vi "SetNag_record_pressure_and_temp.vi"() -> ()   [LabVIEW 2013]
uses:
  <vilib>/Utility/file.llb/Write To Spreadsheet File (string).vi
  <vilib>/Utility/file.llb/Write To Spreadsheet File (DBL).vi
panel:
  out "Read 6":string
  in  "Write 6":string="_STP\r"
  out "Waveform Chart 2":T1(graph)
  out "Read 5":string
  in  "Write 5":string="_TEM\r"
  in  "Write 4":string="_AMB\r"
  out "Read 4":string
  in  "milliseconds to wait":u32=100
  in  "Write 1":string="_OXY\r"
  out "Read 3":string
  in  "Write 3":string="_ETA\r"
  in  "stop 2":bool
  out "Read 2":string
  in  "Write 2":string="_PAB\r"
  out "Read 1":string
  out "Waveform Chart":T2(graph)
  in  "Com Port":i32(ring) items=["Com 1", "Com 2", "Com 3", "Com 4", "Com 5", "Com 6", "COM 7", "COM 8", "COM 9", "COM 10", "COM 11", "COM 12", "com 13", "COM 14"]
  in  "Baud Rate":i32(ring)=2 items=["2400", "4800", "9600", "19200", "38400", "57600", "115200"]
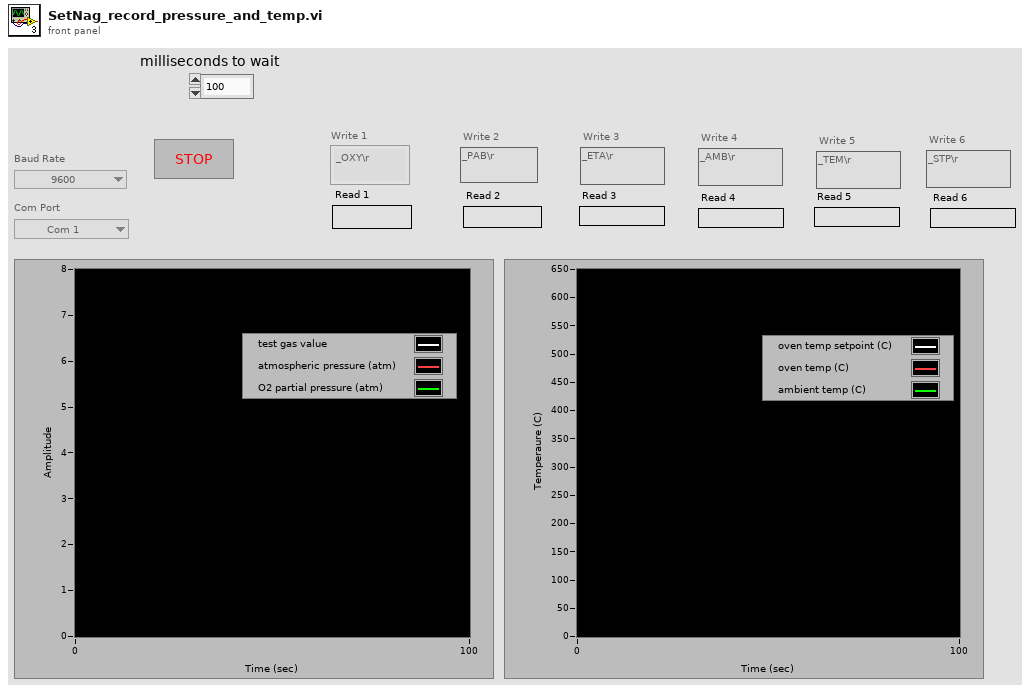
[diagram p1: front panel]
types:
  T1 = cluster{dbl, "string read":dbl, "string read":dbl}
  T2 = cluster{"string read":dbl, "string read":dbl, "string read":dbl}
  T3 = enum16{"no parity", "odd parity", "even parity", "mark parity", "space parity"}
  T4 = cluster{"string read":string, "string read":string, "string read":string}
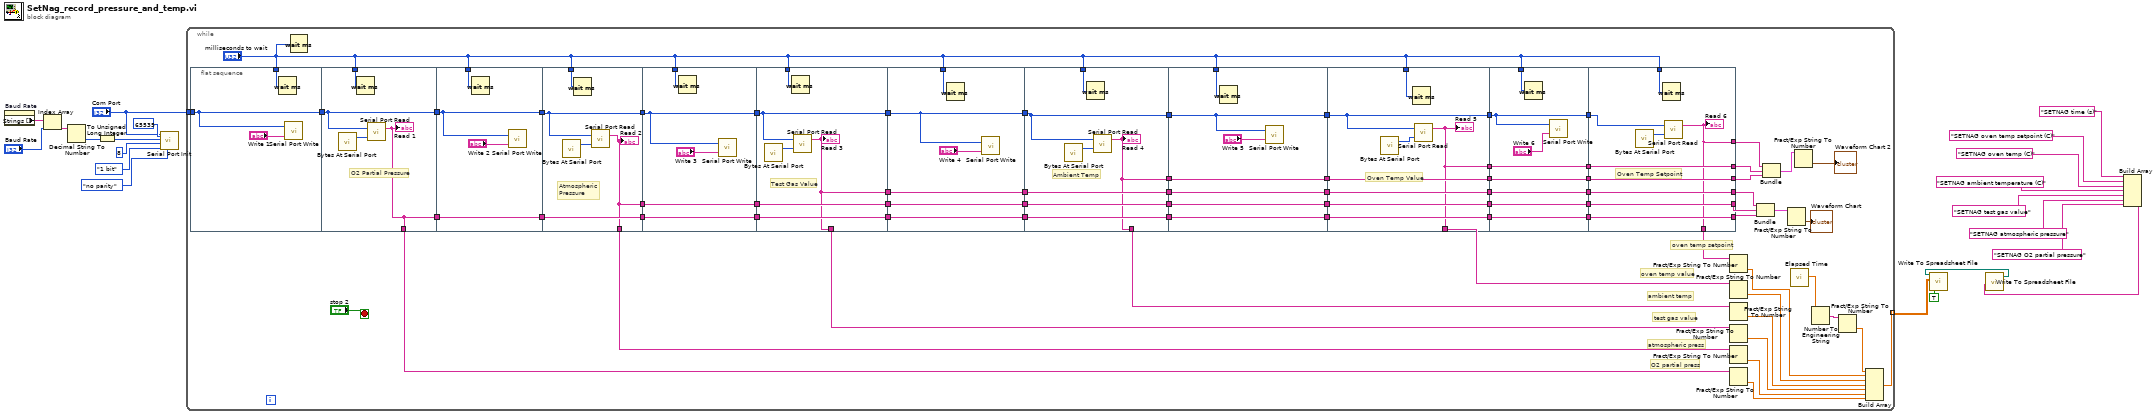
[diagram p0: block diagram]
diagram:
  n1 = property on="Baud Rate" class="Ring (strict)"() -> ("Strings []"=w20:string[])  [unwired: 2 in, 2 out]
  n2 = Index Array(array=w20, index="Baud Rate") -> (element=w19:string)
  n3 = Decimal String To Number(string=w19) -> (number=w21:i32)  [unwired: 2 in, 1 out]
  n4 = To Unsigned Long Integer(number=w21) -> (unsigned 32bit integer=w18:u32)
  n5 = call <vilib>:"Serial Port Init.vi"("parity"=T3."no parity", "buffer size"=u16 65535, "stop bits"=enum16{"1 bit", "1.5 bits", "2 bits"}."1 bit", "data bits"=u16 8, "baud rate"=w18, "port number"="Com Port") -> ()  [unwired: 1 in, 1 out]
  n6 = while {
    tunnel: "Com Port" -> [w88]
    tunnel: [w70] -> w5 mode=indexing
    stop <- "stop 2" stop-if-true
    # "oven temp setpoint"
    # "oven temp value"
    # "ambient temp"
    # "test gas value"
    # "atmospheric press"
    # "O2 partial press"
    n7 = flat-sequence {
      tunnel: w88 -> [w94]
      tunnel: [w94] -> w91
      tunnel: "milliseconds to wait" -> [w92]
      tunnel: w91 -> [w97]
      tunnel: [w97] -> w90
      tunnel: [w96] -> w82
      tunnel: [w96] -> w75
      tunnel: "milliseconds to wait" -> [w95]
      tunnel: [w101] -> w89
      tunnel: w90 -> [w101]
      tunnel: w82 -> [w100]
      tunnel: [w100] -> w81
      tunnel: "milliseconds to wait" -> [w99]
      tunnel: w89 -> [w106]
      tunnel: [w106] -> w86
      tunnel: [w104] -> w84
      tunnel: w81 -> [w105]
      tunnel: [w105] -> w80
      tunnel: [w104] -> w74
      tunnel: "milliseconds to wait" -> [w103]
      tunnel: w86 -> [w111]
      tunnel: [w111] -> w85
      tunnel: w84 -> [w110]
      tunnel: [w110] -> w83
      tunnel: w80 -> [w109]
      tunnel: [w109] -> w79
      tunnel: "milliseconds to wait" -> [w108]
      tunnel: w85 -> [w113]
      tunnel: w83 -> [w117]
      tunnel: w79 -> [w116]
      tunnel: [w115] -> w73
      tunnel: "milliseconds to wait" -> [w114]
      tunnel: [w115] -> w67
      tunnel: [w117] -> w66
      tunnel: [w116] -> w65
      tunnel: [w113] -> w61
      tunnel: w67 -> [w124]
      tunnel: w66 -> [w123]
      tunnel: w65 -> [w122]
      tunnel: [w124] -> w64
      tunnel: [w123] -> w63
      tunnel: [w122] -> w62
      tunnel: w61 -> [w120]
      tunnel: [w120] -> w60
      tunnel: "milliseconds to wait" -> [w119]
      tunnel: w64 -> [w131]
      tunnel: w63 -> [w130]
      tunnel: w62 -> [w129]
      tunnel: w60 -> [w126]
      tunnel: "milliseconds to wait" -> [w127]
      tunnel: [w131] -> w55
      tunnel: [w130] -> w54
      tunnel: [w129] -> w53
      tunnel: [w125] -> w52
      tunnel: [w126] -> w47
      tunnel: [w125] -> w41
      tunnel: w55 -> [w138]
      tunnel: w54 -> [w137]
      tunnel: w53 -> [w136]
      tunnel: w52 -> [w135]
      tunnel: [w138] -> w51
      tunnel: [w137] -> w50
      tunnel: [w136] -> w49
      tunnel: [w135] -> w48
      tunnel: "milliseconds to wait" -> [w134]
      tunnel: w47 -> [w132]
      tunnel: [w132] -> w46
      tunnel: w51 -> [w146]
      tunnel: w50 -> [w145]
      tunnel: w49 -> [w144]
      tunnel: w48 -> [w143]
      tunnel: "milliseconds to wait" -> [w142]
      tunnel: w46 -> [w139]
      tunnel: [w140] -> w40
      tunnel: [w146] -> w39
      tunnel: [w145] -> w38
      tunnel: [w144] -> w37
      tunnel: [w143] -> w36
      tunnel: [w140] -> w35
      tunnel: [w139] -> w28
      tunnel: w39 -> [w154]
      tunnel: w38 -> [w153]
      tunnel: w37 -> [w152]
      tunnel: w36 -> [w151]
      tunnel: w35 -> [w150]
      tunnel: [w154] -> w34
      tunnel: [w153] -> w33
      tunnel: [w152] -> w32
      tunnel: [w151] -> w31
      tunnel: [w150] -> w30
      tunnel: "milliseconds to wait" -> [w148]
      tunnel: w28 -> [w147]
      tunnel: [w147] -> w27
      tunnel: [w159] -> w44
      tunnel: [w160] -> w45
      tunnel: [w161] -> w76
      tunnel: [w162] -> w77
      tunnel: [w163] -> w78
      tunnel: w34 -> [w163]
      tunnel: w33 -> [w162]
      tunnel: w32 -> [w161]
      tunnel: w31 -> [w160]
      tunnel: w30 -> [w159]
      tunnel: "milliseconds to wait" -> [w157]
      tunnel: w27 -> [w156]
      tunnel: [w155] -> w25
      tunnel: [w155] -> w24
      frame #0 {
        n8 = Wait (ms)(milliseconds to wait=w92) -> ()  [unwired: 1 out]
        n9 = call <vilib>:"Serial Port Write.vi"("string to write"="Write 1", "port number"=w94) -> ()  [unwired: 1 out]
      }
      frame #1 {
        # "O2 Partial Pressure"
        n10 = call <vilib>:"Bytes At Serial Port.vi"() -> ("byte count"=w98:u32)  [unwired: 1 in, 1 out]
        n11 = Wait (ms)(milliseconds to wait=w95) -> ()  [unwired: 1 out]
        n12 = call <vilib>:"Serial Port Read.vi"("requested byte count"=w98, "port number"=w97) -> ("string read"=w96:string)  [unwired: 1 out]
        "Read 1" <- w96
      }
      frame #2 {
        n13 = Wait (ms)(milliseconds to wait=w99) -> ()  [unwired: 1 out]
        n14 = call <vilib>:"Serial Port Write.vi"("string to write"="Write 2", "port number"=w101) -> ()  [unwired: 1 out]
      }
      frame #3 {
        # "Atmospheric\nPressure"
        n15 = call <vilib>:"Bytes At Serial Port.vi"() -> ("byte count"=w107:u32)  [unwired: 1 in, 1 out]
        n16 = Wait (ms)(milliseconds to wait=w103) -> ()  [unwired: 1 out]
        n17 = call <vilib>:"Serial Port Read.vi"("requested byte count"=w107, "port number"=w106) -> ("string read"=w104:string)  [unwired: 1 out]
        "Read 2" <- w104
      }
      frame #4 {
        n18 = Wait (ms)(milliseconds to wait=w108) -> ()  [unwired: 1 out]
        n19 = call <vilib>:"Serial Port Write.vi"("string to write"="Write 3", "port number"=w111) -> ()  [unwired: 1 out]
      }
      frame #5 {
        # "Test Gas Value"
        n20 = call <vilib>:"Bytes At Serial Port.vi"() -> ("byte count"=w118:u32)  [unwired: 1 in, 1 out]
        n21 = Wait (ms)(milliseconds to wait=w114) -> ()  [unwired: 1 out]
        n22 = call <vilib>:"Serial Port Read.vi"("requested byte count"=w118, "port number"=w113) -> ("string read"=w115:string)  [unwired: 1 out]
        "Read 3" <- w115
      }
      frame #6 {
        n23 = Wait (ms)(milliseconds to wait=w119) -> ()  [unwired: 1 out]
        n24 = call <vilib>:"Serial Port Write.vi"("string to write"="Write 4", "port number"=w120) -> ()  [unwired: 1 out]
      }
      frame #7 {
        # "Ambient Temp"
        n25 = call <vilib>:"Bytes At Serial Port.vi"() -> ("byte count"=w128:u32)  [unwired: 1 in, 1 out]
        n26 = Wait (ms)(milliseconds to wait=w127) -> ()  [unwired: 1 out]
        n27 = call <vilib>:"Serial Port Read.vi"("requested byte count"=w128, "port number"=w126) -> ("string read"=w125:string)  [unwired: 1 out]
        "Read 4" <- w125
      }
      frame #8 {
        n28 = Wait (ms)(milliseconds to wait=w134) -> ()  [unwired: 1 out]
        n29 = call <vilib>:"Serial Port Write.vi"("string to write"="Write 5", "port number"=w132) -> ()  [unwired: 1 out]
      }
      frame #9 {
        # "Oven Temp Value"
        n30 = call <vilib>:"Bytes At Serial Port.vi"() -> ("byte count"=w141:u32)  [unwired: 1 in, 1 out]
        n31 = Wait (ms)(milliseconds to wait=w142) -> ()  [unwired: 1 out]
        n32 = call <vilib>:"Serial Port Read.vi"("requested byte count"=w141, "port number"=w139) -> ("string read"=w140:string)  [unwired: 1 out]
        "Read 5" <- w140
      }
      frame #10 {
        n33 = Wait (ms)(milliseconds to wait=w148) -> ()  [unwired: 1 out]
        n34 = call <vilib>:"Serial Port Write.vi"("string to write"="Write 6", "port number"=w147) -> ()  [unwired: 1 out]
      }
      frame #11 {
        # "Oven Temp Setpoint"
        n35 = call <vilib>:"Bytes At Serial Port.vi"() -> ("byte count"=w158:u32)  [unwired: 1 in, 1 out]
        n36 = Wait (ms)(milliseconds to wait=w157) -> ()  [unwired: 1 out]
        n37 = call <vilib>:"Serial Port Read.vi"("requested byte count"=w158, "port number"=w156) -> ("string read"=w155:string)  [unwired: 1 out]
        "Read 6" <- w155
      }
    }
    n38 = Wait (ms)(milliseconds to wait="milliseconds to wait") -> ()  [unwired: 1 out]
    n39 = Fract/Exp String To Number(string=w24) -> (number=w23:dbl)  [unwired: 3 in, 1 out]
    n40 = Fract/Exp String To Number(string=w40) -> (number=w42:dbl)  [unwired: 3 in, 1 out]
    n41 = Fract/Exp String To Number(string=w41) -> (number=w56:dbl)  [unwired: 3 in, 1 out]
    n42 = Fract/Exp String To Number(string=w73) -> (number=w57:dbl)  [unwired: 3 in, 1 out]
    n43 = Fract/Exp String To Number(string=w74) -> (number=w58:dbl)  [unwired: 3 in, 1 out]
    n44 = Fract/Exp String To Number(string=w75) -> (number=w59:dbl)  [unwired: 3 in, 1 out]
    n45 = Bundle("string read"=w78, "string read"=w77, "string read"=w76) -> (w69:T4)  [unwired: 1 in]
    n46 = Bundle("string read"=w25, "string read"=w44, "string read"=w45) -> (w26:T4)  [unwired: 1 in]
    n47 = Fract/Exp String To Number(string=w69) -> (number=→"Waveform Chart":T2)  [unwired: 3 in, 1 out]
    n48 = call "Elapsed Time"() -> ("Elapsed Time (s)"=w72:dbl)  [unwired: 12 in, 7 out]
    n49 = Fract/Exp String To Number(string=w26) -> (number=→"Waveform Chart 2":T2)  [unwired: 3 in, 1 out]
    n50 = Number To Engineering String(4:w72) -> (0:w71:string)  [unwired: 3 in]
    n51 = Fract/Exp String To Number(string=w71) -> (number=w22:dbl)  [unwired: 3 in, 1 out]
    n52 = Build Array(w22, w23, w42, w56, w57, w58, w59) -> (w70:dbl[])
  }
  n53 = Build Array("SETNAG time (s)", "SETNAG oven temp setpoint (C)", "SETNAG oven temp (C)", "SETNAG ambient temperature (C)", "SETNAG test gas value", "SETNAG atmospheric pressure", "SETNAG O2 partial pressure") -> (w9:string[])
  n54 = call-poly <vilib>:"Write To Spreadsheet File.vi"("1D data"=w9) -> ("new file path (Not A Path if cancelled)"=w11:path)  [unwired: 7 in]
  n55 = call-poly <vilib>:"Write To Spreadsheet File.vi"("append to file? (new file:F)"=TRUE, "2D data"=w5, "file path (dialog if empty)"=w11) -> ()  [unwired: 5 in, 1 out]
